vi "Check.vi"(11 "Point to Check":cluster{i64, i64, i64}) -> (3 "response":T1)   [LabVIEW 2021, in "d18.lvlib"]
uses:
  d18.lvlib
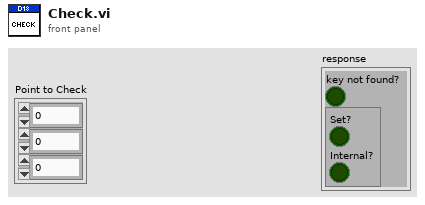
[diagram p1: front panel]
types:
  T1 = cluster{"key not found?":bool, cluster{"Set?":bool, "Internal?":bool}}
  T2 = cluster{"Point to Check":cluster{i64, i64, i64}, "notifier out":refnum<notifier>}
  T3 = cluster{string, cluster{"Point to Check":cluster{i64, i64, i64}, "notifier out":refnum<notifier>}}
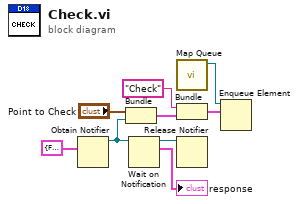
[diagram p0: block diagram]
diagram:
  n1 = Obtain Notifier(notification data type=T1 {"key not found?"=FALSE, {"Set?"=FALSE, "Internal?"=FALSE}} ("output cluster")) -> (notifier out=w7:refnum<notifier>)  [unwired: 3 in, 2 out]
  n2 = Bundle("Point to Check"="Point to Check", "notifier out"=w7) -> (w5:T2)  [unwired: 1 in]
  n3 = Wait on Notification(notifier=w7) -> (notifier out=w8:refnum<notifier>, notification=→"response":T1)  [unwired: 3 in, 2 out]
  n4 = call "Map Queue.vi"() -> ("Queue out"=w2:refnum<queue>)  [unwired: 11 in]
  n5 = Bundle("Check", w5) -> (w3:T3)  [unwired: 1 in]
  n6 = Release Notifier(notifier=w8) -> ()  [unwired: 2 in, 3 out]
  n7 = Enqueue Element(queue=w2, element=w3) -> ()  [unwired: 2 in, 3 out]
